vi "PicoScope6000aSettings.vi"(0 "handle in":i16, 1 "Device Info":T3, 2 "Channels":T2 {"Channel H Settings"."BandWidth" items=["Full", "100kHz", "20kHz", "1MHz", "20MHz", "25MHz", "50MHz", "200MHz", "250MHz", "500MHz"]; "Channel H Settings"."Range" items=["10mV", "20mV", "50mV", "100mV", "200mV", "500mV", "1V", "2V", "5V", "10V", "20V", "50V", "100V", "200V", "x10_Probe_100mV", "x10_Probe_200mV", "x10_Probe_500mV", "x10_Probe_1V", "x10_Probe_2V", "x10_Probe_5V", "x10_Probe_10V", "x10_Probe_20V", "x10_Probe_50V", "x10_Probe_100V", "x10_Probe_200V", "x10_Probe_500V", "CURRENT_CLAMP_60A_2A", "CURRENT_CLAMP_60A_5A", "CURRENT_CLAMP_60A_10A", "CURRENT_CLAMP_60A_20A", "CURRENT_CLAMP_60A_50A", "CURRENT_CLAMP_60A_60A", "CURRENT_CLAMP_60A_V2_0_5A", "CURRENT_CLAMP_60A_V2_1A", "CURRENT_CLAMP_60A_V2_2A", "CURRENT_CLAMP_60A_V2_5A", "CURRENT_CLAMP_60A_V2_10A", "CURRENT_CLAMP_60A_V2_20A", "CURRENT_CLAMP_60A_V2_50A", "CURRENT_CLAMP_60A_V2_60A", "RESISTANCE_LEAD_NEG5_TO_20OHM", "RESISTANCE_LEAD_NEG50_TO_200OHM", "RESISTANCE_LEAD_NEG500_TO_2KOHM", "RESISTANCE_LEAD_NEG5K_TO_20KOHM", "RESISTANCE_LEAD_NEG50K_TO_LEAD_200KOHM", "RESISTANCE_LEAD_NEG500K_TO_LEAD_2MOHM", "RESISTANCE_LEAD_DIODE_TEST", "HT_NEG3_TO_5KV", "HT_NEG3_TO_10KV", "HT_NEG5_TO_20KV", "HT_NEG5_TO_50KV", "HT_NEG5_TO_100KV", "HT_NEG3_TO_5KV_INVERTED", "HT_NEG3_TO_10KV_INVERTED", "HT_NEG5_TO_20KV_INVERTED", "HT_NEG5_TO_50KV_INVERTED", "HT_NEG5_TO_100KV_INVERTED", "TEMPERATURE_NEG50_TO_150DEGC", "PRESSURE_SENSOR_-100k-150k_PASCALS", "PRESSURE_SENSOR_-100k_TO_400k_PASCALS", "PRESSURE_SENSOR_-200k_TO_800k_PASCALS", "PRESSURE_SENSOR_-400k_TO_1600k_PASCALS", "PRESSURE_SENSOR_-400k_TO_3400k_PASCALS", "PRESSURE_SENSOR_-150k_TO_1350k_PASCALS"]; "Channel H Settings"."Coupling" items=["AC", "DC 1M Ohm", "DC 50 Ohm"]; "Channel G Settings"."BandWidth" items=["Full", "100kHz", "20kHz", "1MHz", "20MHz", "25MHz", "50MHz", "200MHz", "250MHz", "500MHz"]; "Channel G Settings"."Range" items=["10mV", "20mV", "50mV", "100mV", "200mV", "500mV", "1V", "2V", "5V", "10V", "20V", "50V", "100V", "200V", "x10_Probe_100mV", "x10_Probe_200mV", "x10_Probe_500mV", "x10_Probe_1V", "x10_Probe_2V", "x10_Probe_5V", "x10_Probe_10V", "x10_Probe_20V", "x10_Probe_50V", "x10_Probe_100V", "x10_Probe_200V", "x10_Probe_500V", "CURRENT_CLAMP_60A_2A", "CURRENT_CLAMP_60A_5A", "CURRENT_CLAMP_60A_10A", "CURRENT_CLAMP_60A_20A", "CURRENT_CLAMP_60A_50A", "CURRENT_CLAMP_60A_60A", "CURRENT_CLAMP_60A_V2_0_5A", "CURRENT_CLAMP_60A_V2_1A", "CURRENT_CLAMP_60A_V2_2A", "CURRENT_CLAMP_60A_V2_5A", "CURRENT_CLAMP_60A_V2_10A", "CURRENT_CLAMP_60A_V2_20A", "CURRENT_CLAMP_60A_V2_50A", "CURRENT_CLAMP_60A_V2_60A", "RESISTANCE_LEAD_NEG5_TO_20OHM", "RESISTANCE_LEAD_NEG50_TO_200OHM", "RESISTANCE_LEAD_NEG500_TO_2KOHM", "RESISTANCE_LEAD_NEG5K_TO_20KOHM", "RESISTANCE_LEAD_NEG50K_TO_LEAD_200KOHM", "RESISTANCE_LEAD_NEG500K_TO_LEAD_2MOHM", "RESISTANCE_LEAD_DIODE_TEST", "HT_NEG3_TO_5KV", "HT_NEG3_TO_10KV", "HT_NEG5_TO_20KV", "HT_NEG5_TO_50KV", "HT_NEG5_TO_100KV", "HT_NEG3_TO_5KV_INVERTED", "HT_NEG3_TO_10KV_INVERTED", "HT_NEG5_TO_20KV_INVERTED", "HT_NEG5_TO_50KV_INVERTED", "HT_NEG5_TO_100KV_INVERTED", "TEMPERATURE_NEG50_TO_150DEGC", "PRESSURE_SENSOR_-100k-150k_PASCALS", "PRESSURE_SENSOR_-100k_TO_400k_PASCALS", "PRESSURE_SENSOR_-200k_TO_800k_PASCALS", "PRESSURE_SENSOR_-400k_TO_1600k_PASCALS", "PRESSURE_SENSOR_-400k_TO_3400k_PASCALS", "PRESSURE_SENSOR_-150k_TO_1350k_PASCALS"]; "Channel G Settings"."Coupling" items=["AC", "DC 1M Ohm", "DC 50 Ohm"]; "Channel F Settings"."BandWidth" items=["Full", "100kHz", "20kHz", "1MHz", "20MHz", "25MHz", "50MHz", "200MHz", "250MHz", "500MHz"]; "Channel F Settings"."Range" items=["10mV", "20mV", "50mV", "100mV", "200mV", "500mV", "1V", "2V", "5V", "10V", "20V", "50V", "100V", "200V", "x10_Probe_100mV", "x10_Probe_200mV", "x10_Probe_500mV", "x10_Probe_1V", "x10_Probe_2V", "x10_Probe_5V", "x10_Probe_10V", "x10_Probe_20V", "x10_Probe_50V", "x10_Probe_100V", "x10_Probe_200V", "x10_Probe_500V", "CURRENT_CLAMP_60A_2A", "CURRENT_CLAMP_60A_5A", "CURRENT_CLAMP_60A_10A", "CURRENT_CLAMP_60A_20A", "CURRENT_CLAMP_60A_50A", "CURRENT_CLAMP_60A_60A", "CURRENT_CLAMP_60A_V2_0_5A", "CURRENT_CLAMP_60A_V2_1A", "CURRENT_CLAMP_60A_V2_2A", "CURRENT_CLAMP_60A_V2_5A", "CURRENT_CLAMP_60A_V2_10A", "CURRENT_CLAMP_60A_V2_20A", "CURRENT_CLAMP_60A_V2_50A", "CURRENT_CLAMP_60A_V2_60A", "RESISTANCE_LEAD_NEG5_TO_20OHM", "RESISTANCE_LEAD_NEG50_TO_200OHM", "RESISTANCE_LEAD_NEG500_TO_2KOHM", "RESISTANCE_LEAD_NEG5K_TO_20KOHM", "RESISTANCE_LEAD_NEG50K_TO_LEAD_200KOHM", "RESISTANCE_LEAD_NEG500K_TO_LEAD_2MOHM", "RESISTANCE_LEAD_DIODE_TEST", "HT_NEG3_TO_5KV", "HT_NEG3_TO_10KV", "HT_NEG5_TO_20KV", "HT_NEG5_TO_50KV", "HT_NEG5_TO_100KV", "HT_NEG3_TO_5KV_INVERTED", "HT_NEG3_TO_10KV_INVERTED", "HT_NEG5_TO_20KV_INVERTED", "HT_NEG5_TO_50KV_INVERTED", "HT_NEG5_TO_100KV_INVERTED", "TEMPERATURE_NEG50_TO_150DEGC", "PRESSURE_SENSOR_-100k-150k_PASCALS", "PRESSURE_SENSOR_-100k_TO_400k_PASCALS", "PRESSURE_SENSOR_-200k_TO_800k_PASCALS", "PRESSURE_SENSOR_-400k_TO_1600k_PASCALS", "PRESSURE_SENSOR_-400k_TO_3400k_PASCALS", "PRESSURE_SENSOR_-150k_TO_1350k_PASCALS"]; "Channel F Settings"."Coupling" items=["AC", "DC 1M Ohm", "DC 50 Ohm"]; "Channel E Settings"."BandWidth" items=["Full", "100kHz", "20kHz", "1MHz", "20MHz", "25MHz", "50MHz", "200MHz", "250MHz", "500MHz"]; "Channel E Settings"."Range" items=["10mV", "20mV", "50mV", "100mV", "200mV", "500mV", "1V", "2V", "5V", "10V", "20V", "50V", "100V", "200V", "x10_Probe_100mV", "x10_Probe_200mV", "x10_Probe_500mV", "x10_Probe_1V", "x10_Probe_2V", "x10_Probe_5V", "x10_Probe_10V", "x10_Probe_20V", "x10_Probe_50V", "x10_Probe_100V", "x10_Probe_200V", "x10_Probe_500V", "CURRENT_CLAMP_60A_2A", "CURRENT_CLAMP_60A_5A", "CURRENT_CLAMP_60A_10A", "CURRENT_CLAMP_60A_20A", "CURRENT_CLAMP_60A_50A", "CURRENT_CLAMP_60A_60A", "CURRENT_CLAMP_60A_V2_0_5A", "CURRENT_CLAMP_60A_V2_1A", "CURRENT_CLAMP_60A_V2_2A", "CURRENT_CLAMP_60A_V2_5A", "CURRENT_CLAMP_60A_V2_10A", "CURRENT_CLAMP_60A_V2_20A", "CURRENT_CLAMP_60A_V2_50A", "CURRENT_CLAMP_60A_V2_60A", "RESISTANCE_LEAD_NEG5_TO_20OHM", "RESISTANCE_LEAD_NEG50_TO_200OHM", "RESISTANCE_LEAD_NEG500_TO_2KOHM", "RESISTANCE_LEAD_NEG5K_TO_20KOHM", "RESISTANCE_LEAD_NEG50K_TO_LEAD_200KOHM", "RESISTANCE_LEAD_NEG500K_TO_LEAD_2MOHM", "RESISTANCE_LEAD_DIODE_TEST", "HT_NEG3_TO_5KV", "HT_NEG3_TO_10KV", "HT_NEG5_TO_20KV", "HT_NEG5_TO_50KV", "HT_NEG5_TO_100KV", "HT_NEG3_TO_5KV_INVERTED", "HT_NEG3_TO_10KV_INVERTED", "HT_NEG5_TO_20KV_INVERTED", "HT_NEG5_TO_50KV_INVERTED", "HT_NEG5_TO_100KV_INVERTED", "TEMPERATURE_NEG50_TO_150DEGC", "PRESSURE_SENSOR_-100k-150k_PASCALS", "PRESSURE_SENSOR_-100k_TO_400k_PASCALS", "PRESSURE_SENSOR_-200k_TO_800k_PASCALS", "PRESSURE_SENSOR_-400k_TO_1600k_PASCALS", "PRESSURE_SENSOR_-400k_TO_3400k_PASCALS", "PRESSURE_SENSOR_-150k_TO_1350k_PASCALS"]; "Channel E Settings"."Coupling" items=["AC", "DC 1M Ohm", "DC 50 Ohm"]; "Channel D Settings"."BandWidth" items=["Full", "100kHz", "20kHz", "1MHz", "20MHz", "25MHz", "50MHz", "200MHz", "250MHz", "500MHz"]; "Channel D Settings"."Range" items=["10mV", "20mV", "50mV", "100mV", "200mV", "500mV", "1V", "2V", "5V", "10V", "20V", "50V", "100V", "200V", "x10_Probe_100mV", "x10_Probe_200mV", "x10_Probe_500mV", "x10_Probe_1V", "x10_Probe_2V", "x10_Probe_5V", "x10_Probe_10V", "x10_Probe_20V", "x10_Probe_50V", "x10_Probe_100V", "x10_Probe_200V", "x10_Probe_500V", "CURRENT_CLAMP_60A_2A", "CURRENT_CLAMP_60A_5A", "CURRENT_CLAMP_60A_10A", "CURRENT_CLAMP_60A_20A", "CURRENT_CLAMP_60A_50A", "CURRENT_CLAMP_60A_60A", "CURRENT_CLAMP_60A_V2_0_5A", "CURRENT_CLAMP_60A_V2_1A", "CURRENT_CLAMP_60A_V2_2A", "CURRENT_CLAMP_60A_V2_5A", "CURRENT_CLAMP_60A_V2_10A", "CURRENT_CLAMP_60A_V2_20A", "CURRENT_CLAMP_60A_V2_50A", "CURRENT_CLAMP_60A_V2_60A", "RESISTANCE_LEAD_NEG5_TO_20OHM", "RESISTANCE_LEAD_NEG50_TO_200OHM", "RESISTANCE_LEAD_NEG500_TO_2KOHM", "RESISTANCE_LEAD_NEG5K_TO_20KOHM", "RESISTANCE_LEAD_NEG50K_TO_LEAD_200KOHM", "RESISTANCE_LEAD_NEG500K_TO_LEAD_2MOHM", "RESISTANCE_LEAD_DIODE_TEST", "HT_NEG3_TO_5KV", "HT_NEG3_TO_10KV", "HT_NEG5_TO_20KV", "HT_NEG5_TO_50KV", "HT_NEG5_TO_100KV", "HT_NEG3_TO_5KV_INVERTED", "HT_NEG3_TO_10KV_INVERTED", "HT_NEG5_TO_20KV_INVERTED", "HT_NEG5_TO_50KV_INVERTED", "HT_NEG5_TO_100KV_INVERTED", "TEMPERATURE_NEG50_TO_150DEGC", "PRESSURE_SENSOR_-100k-150k_PASCALS", "PRESSURE_SENSOR_-100k_TO_400k_PASCALS", "PRESSURE_SENSOR_-200k_TO_800k_PASCALS", "PRESSURE_SENSOR_-400k_TO_1600k_PASCALS", "PRESSURE_SENSOR_-400k_TO_3400k_PASCALS", "PRESSURE_SENSOR_-150k_TO_1350k_PASCALS"]; "Channel D Settings"."Coupling" items=["AC", "DC 1M Ohm", "DC 50 Ohm"]; "Channel C Settings"."BandWidth" items=["Full", "100kHz", "20kHz", "1MHz", "20MHz", "25MHz", "50MHz", "200MHz", "250MHz", "500MHz"]; "Channel C Settings"."Range" items=["10mV", "20mV", "50mV", "100mV", "200mV", "500mV", "1V", "2V", "5V", "10V", "20V", "50V", "100V", "200V", "x10_Probe_100mV", "x10_Probe_200mV", "x10_Probe_500mV", "x10_Probe_1V", "x10_Probe_2V", "x10_Probe_5V", "x10_Probe_10V", "x10_Probe_20V", "x10_Probe_50V", "x10_Probe_100V", "x10_Probe_200V", "x10_Probe_500V", "CURRENT_CLAMP_60A_2A", "CURRENT_CLAMP_60A_5A", "CURRENT_CLAMP_60A_10A", "CURRENT_CLAMP_60A_20A", "CURRENT_CLAMP_60A_50A", "CURRENT_CLAMP_60A_60A", "CURRENT_CLAMP_60A_V2_0_5A", "CURRENT_CLAMP_60A_V2_1A", "CURRENT_CLAMP_60A_V2_2A", "CURRENT_CLAMP_60A_V2_5A", "CURRENT_CLAMP_60A_V2_10A", "CURRENT_CLAMP_60A_V2_20A", "CURRENT_CLAMP_60A_V2_50A", "CURRENT_CLAMP_60A_V2_60A", "RESISTANCE_LEAD_NEG5_TO_20OHM", "RESISTANCE_LEAD_NEG50_TO_200OHM", "RESISTANCE_LEAD_NEG500_TO_2KOHM", "RESISTANCE_LEAD_NEG5K_TO_20KOHM", "RESISTANCE_LEAD_NEG50K_TO_LEAD_200KOHM", "RESISTANCE_LEAD_NEG500K_TO_LEAD_2MOHM", "RESISTANCE_LEAD_DIODE_TEST", "HT_NEG3_TO_5KV", "HT_NEG3_TO_10KV", "HT_NEG5_TO_20KV", "HT_NEG5_TO_50KV", "HT_NEG5_TO_100KV", "HT_NEG3_TO_5KV_INVERTED", "HT_NEG3_TO_10KV_INVERTED", "HT_NEG5_TO_20KV_INVERTED", "HT_NEG5_TO_50KV_INVERTED", "HT_NEG5_TO_100KV_INVERTED", "TEMPERATURE_NEG50_TO_150DEGC", "PRESSURE_SENSOR_-100k-150k_PASCALS", "PRESSURE_SENSOR_-100k_TO_400k_PASCALS", "PRESSURE_SENSOR_-200k_TO_800k_PASCALS", "PRESSURE_SENSOR_-400k_TO_1600k_PASCALS", "PRESSURE_SENSOR_-400k_TO_3400k_PASCALS", "PRESSURE_SENSOR_-150k_TO_1350k_PASCALS"]; "Channel C Settings"."Coupling" items=["AC", "DC 1M Ohm", "DC 50 Ohm"]; "Channel B Settings"."BandWidth" items=["Full", "100kHz", "20kHz", "1MHz", "20MHz", "25MHz", "50MHz", "200MHz", "250MHz", "500MHz"]; "Channel B Settings"."Range" items=["10mV", "20mV", "50mV", "100mV", "200mV", "500mV", "1V", "2V", "5V", "10V", "20V", "50V", "100V", "200V", "x10_Probe_100mV", "x10_Probe_200mV", "x10_Probe_500mV", "x10_Probe_1V", "x10_Probe_2V", "x10_Probe_5V", "x10_Probe_10V", "x10_Probe_20V", "x10_Probe_50V", "x10_Probe_100V", "x10_Probe_200V", "x10_Probe_500V", "CURRENT_CLAMP_60A_2A", "CURRENT_CLAMP_60A_5A", "CURRENT_CLAMP_60A_10A", "CURRENT_CLAMP_60A_20A", "CURRENT_CLAMP_60A_50A", "CURRENT_CLAMP_60A_60A", "CURRENT_CLAMP_60A_V2_0_5A", "CURRENT_CLAMP_60A_V2_1A", "CURRENT_CLAMP_60A_V2_2A", "CURRENT_CLAMP_60A_V2_5A", "CURRENT_CLAMP_60A_V2_10A", "CURRENT_CLAMP_60A_V2_20A", "CURRENT_CLAMP_60A_V2_50A", "CURRENT_CLAMP_60A_V2_60A", "RESISTANCE_LEAD_NEG5_TO_20OHM", "RESISTANCE_LEAD_NEG50_TO_200OHM", "RESISTANCE_LEAD_NEG500_TO_2KOHM", "RESISTANCE_LEAD_NEG5K_TO_20KOHM", "RESISTANCE_LEAD_NEG50K_TO_LEAD_200KOHM", "RESISTANCE_LEAD_NEG500K_TO_LEAD_2MOHM", "RESISTANCE_LEAD_DIODE_TEST", "HT_NEG3_TO_5KV", "HT_NEG3_TO_10KV", "HT_NEG5_TO_20KV", "HT_NEG5_TO_50KV", "HT_NEG5_TO_100KV", "HT_NEG3_TO_5KV_INVERTED", "HT_NEG3_TO_10KV_INVERTED", "HT_NEG5_TO_20KV_INVERTED", "HT_NEG5_TO_50KV_INVERTED", "HT_NEG5_TO_100KV_INVERTED", "TEMPERATURE_NEG50_TO_150DEGC", "PRESSURE_SENSOR_-100k-150k_PASCALS", "PRESSURE_SENSOR_-100k_TO_400k_PASCALS", "PRESSURE_SENSOR_-200k_TO_800k_PASCALS", "PRESSURE_SENSOR_-400k_TO_1600k_PASCALS", "PRESSURE_SENSOR_-400k_TO_3400k_PASCALS", "PRESSURE_SENSOR_-150k_TO_1350k_PASCALS"]; "Channel B Settings"."Coupling" items=["AC", "DC 1M Ohm", "DC 50 Ohm"]; "Channel A Settings"."Range" items=["10mV", "20mV", "50mV", "100mV", "200mV", "500mV", "1V", "2V", "5V", "10V", "20V", "50V", "100V", "200V", "x10_Probe_100mV", "x10_Probe_200mV", "x10_Probe_500mV", "x10_Probe_1V", "x10_Probe_2V", "x10_Probe_5V", "x10_Probe_10V", "x10_Probe_20V", "x10_Probe_50V", "x10_Probe_100V", "x10_Probe_200V", "x10_Probe_500V", "CURRENT_CLAMP_60A_2A", "CURRENT_CLAMP_60A_5A", "CURRENT_CLAMP_60A_10A", "CURRENT_CLAMP_60A_20A", "CURRENT_CLAMP_60A_50A", "CURRENT_CLAMP_60A_60A", "CURRENT_CLAMP_60A_V2_0_5A", "CURRENT_CLAMP_60A_V2_1A", "CURRENT_CLAMP_60A_V2_2A", "CURRENT_CLAMP_60A_V2_5A", "CURRENT_CLAMP_60A_V2_10A", "CURRENT_CLAMP_60A_V2_20A", "CURRENT_CLAMP_60A_V2_50A", "CURRENT_CLAMP_60A_V2_60A", "RESISTANCE_LEAD_NEG5_TO_20OHM", "RESISTANCE_LEAD_NEG50_TO_200OHM", "RESISTANCE_LEAD_NEG500_TO_2KOHM", "RESISTANCE_LEAD_NEG5K_TO_20KOHM", "RESISTANCE_LEAD_NEG50K_TO_LEAD_200KOHM", "RESISTANCE_LEAD_NEG500K_TO_LEAD_2MOHM", "RESISTANCE_LEAD_DIODE_TEST", "HT_NEG3_TO_5KV", "HT_NEG3_TO_10KV", "HT_NEG5_TO_20KV", "HT_NEG5_TO_50KV", "HT_NEG5_TO_100KV", "HT_NEG3_TO_5KV_INVERTED", "HT_NEG3_TO_10KV_INVERTED", "HT_NEG5_TO_20KV_INVERTED", "HT_NEG5_TO_50KV_INVERTED", "HT_NEG5_TO_100KV_INVERTED", "TEMPERATURE_NEG50_TO_150DEGC", "PRESSURE_SENSOR_-100k-150k_PASCALS", "PRESSURE_SENSOR_-100k_TO_400k_PASCALS", "PRESSURE_SENSOR_-200k_TO_800k_PASCALS", "PRESSURE_SENSOR_-400k_TO_1600k_PASCALS", "PRESSURE_SENSOR_-400k_TO_3400k_PASCALS", "PRESSURE_SENSOR_-150k_TO_1350k_PASCALS"]; "Channel A Settings"."BandWidth" items=["Full", "100kHz", "20kHz", "1MHz", "20MHz", "25MHz", "50MHz", "200MHz", "250MHz", "500MHz"]; "Channel A Settings"."Coupling" items=["AC", "DC 1M Ohm", "DC 50 Ohm"]}, 7 "Max ADC value":i16, 11 "error in (no error)":errorcluster, 12 "Trigger Settings":T4 {"Trigger Source" items=["Channel A", "Channel B", "Channel C", "Channel D", "Channel E", "Channel F", "Channel G", "Channel H", "Port 0", "Port 1", "Trigger AUX"]; "Trigger Direction" items=["Above", "Below", "Rising", "Falling", "Rising or Falling"]; "Trigger Threshold (Volts/Probe Units)" format="%#_6p"}, 14 "Digital Channels":T1 {"Port 1 Settings"."Threshold Level (Volts)" format="%#_4p"; "Port 1 Settings"."Hysteresis" items=["PICO_VERY_HIGH_400MV", "PICO_HIGH_200MV", "PICO_NORMAL_100MV", "PICO_LOW_50MV"]; "Port 0 Settings"."Threshold Level (Volts)" format="%#_4p"; "Port 0 Settings"."Hysteresis" items=["PICO_VERY_HIGH_400MV", "PICO_HIGH_200MV", "PICO_NORMAL_100MV", "PICO_LOW_50MV"]}) -> (3 "Enabled array":i16[](array[numeric]), 4 "handle out":i16, 15 "error out":errorcluster)   [LabVIEW 2009]
doc: "Sets up channels and calls setSimpleTrigger"
uses:
  ps6000a.dll
  PicoScope6000aAnalogChannelSettings.ctl
  PicoScope6000aDigitalChannelSettings.ctl
panel:
  # "D8-D15"
  # "DO-D7"
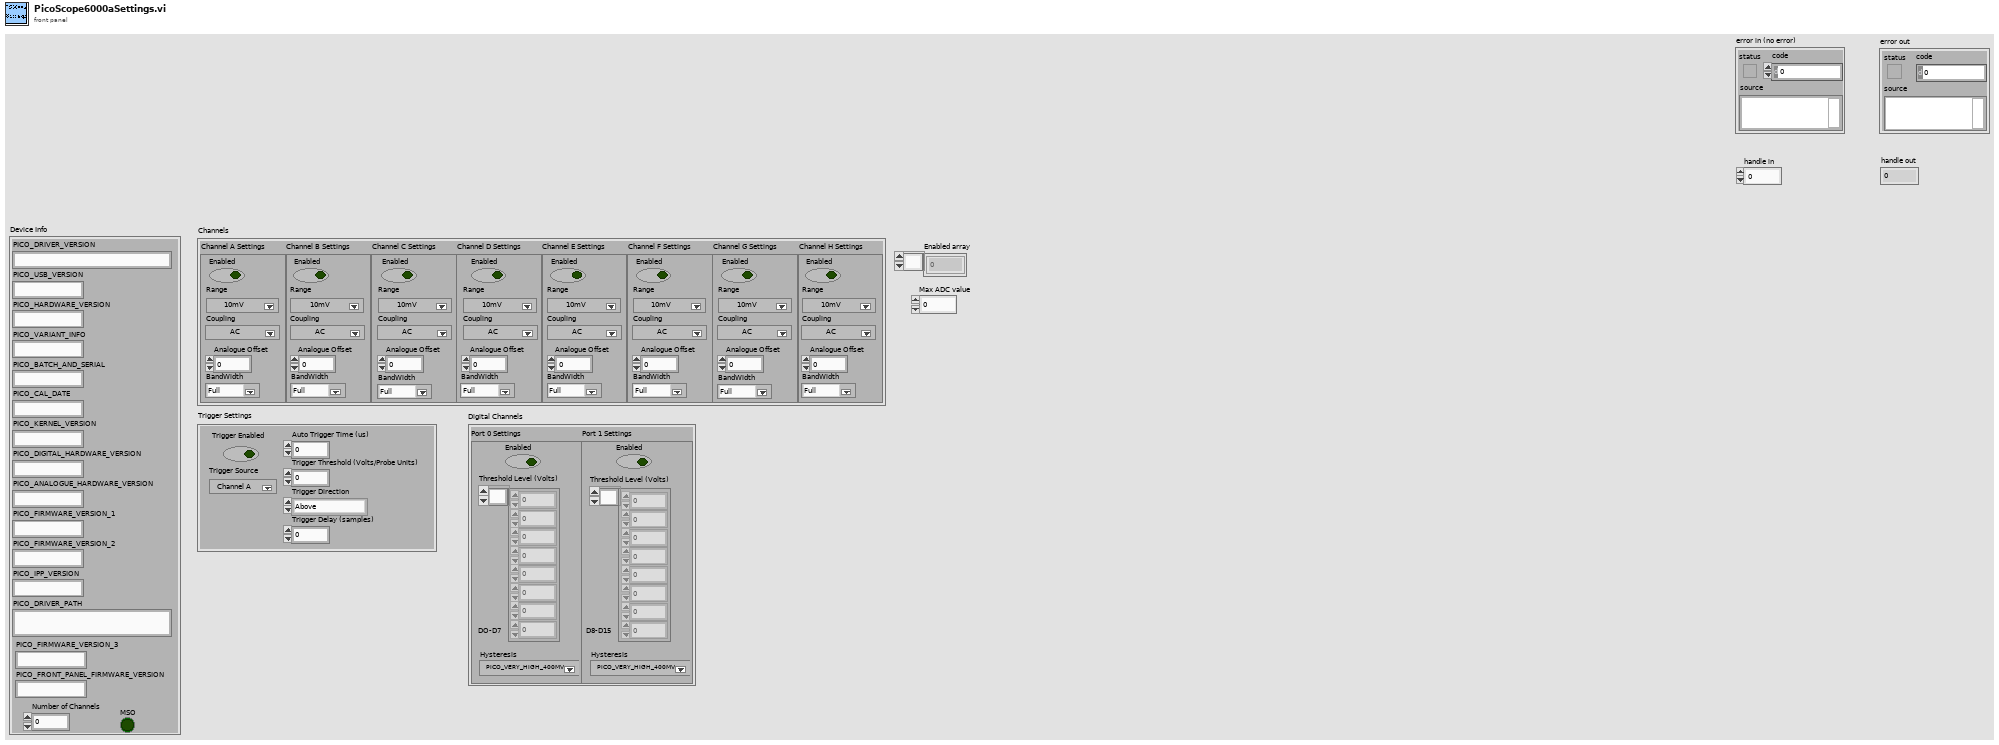
[diagram p1: front panel]
types:
  T1 = typedef "PicoScope6000aDigitalChannelSettings.ctl" = cluster{"Port 0 Settings ":cluster{"Enabled":bool, "Hysteresis":u32, "Threshold Level (Volts)":dbl[]}, "Port 1 Settings":cluster{"Enabled":bool, "Hysteresis":u32, "Threshold Level (Volts)":dbl[]}}
  T2 = typedef "PicoScope6000aAnalogChannelSettings.ctl" = cluster{"Channel A Settings ":cluster{"Enabled":bool, "Coupling":i16, "Range":u16, "Analogue Offset":dbl, "BandWidth":u32}, "Channel B Settings ":cluster{"Enabled":bool, "Coupling":i16, "Range":u16, "Analogue Offset":dbl, "BandWidth":u32}, "Channel C Settings ":cluster{"Enabled":bool, "Coupling":i16, "Range":u16, "Analogue Offset":dbl, "BandWidth":u32}, "Channel D Settings ":cluster{"Enabled":bool, "Coupling":i16, "Range":u16, "Analogue Offset":dbl, "BandWidth":u32}, "Channel E Settings ":cluster{"Enabled":bool, "Coupling":i16, "Range":u16, "Analogue Offset":dbl, "BandWidth":u32}, "Channel F Settings ":cluster{"Enabled":bool, "Coupling":i16, "Range":u16, "Analogue Offset":dbl, "BandWidth":u32}, "Channel G Settings ":cluster{"Enabled":bool, "Coupling":i16, "Range":u16, "Analogue Offset":dbl, "BandWidth":u32}, "Channel H Settings ":cluster{"Enabled":bool, "Coupling":i16, "Range":u16, "Analogue Offset":dbl, "BandWidth":u32}}
  T3 = cluster{"PICO_DRIVER_VERSION":string, "PICO_USB_VERSION":string, "PICO_HARDWARE_VERSION":string, "PICO_VARIANT_INFO":string, "PICO_BATCH_AND_SERIAL":string, "PICO_CAL_DATE":string, "PICO_KERNEL_VERSION":string, "PICO_DIGITAL_HARDWARE_VERSION":string, "PICO_ANALOGUE_HARDWARE_VERSION":string, "PICO_FIRMWARE_VERSION_1":string, "PICO_FIRMWARE_VERSION_2":string, "PICO_IPP_VERSION":string, "PICO_DRIVER_PATH":string, "PICO_FIRMWARE_VERSION_3":string, "PICO_FRONT_PANEL_FIRMWARE_VERSION":string, "Number of Channels":i16, "MSO":bool}
  T4 = cluster{"Trigger Enabled":bool, "Trigger Threshold (Volts/Probe Units)":dbl, "Trigger Direction":u16, "Trigger Delay (samples)":u64, "Auto Trigger Time (us)":u32, "Trigger Source":u32}
  T5 = cluster{"Enabled":bool, "Coupling":i16, "Range":u16, "Analogue Offset":dbl, "BandWidth":u32}
  T6 = cluster{"Enabled":bool, "Hysteresis":u32, "Threshold Level (Volts)":dbl[]}
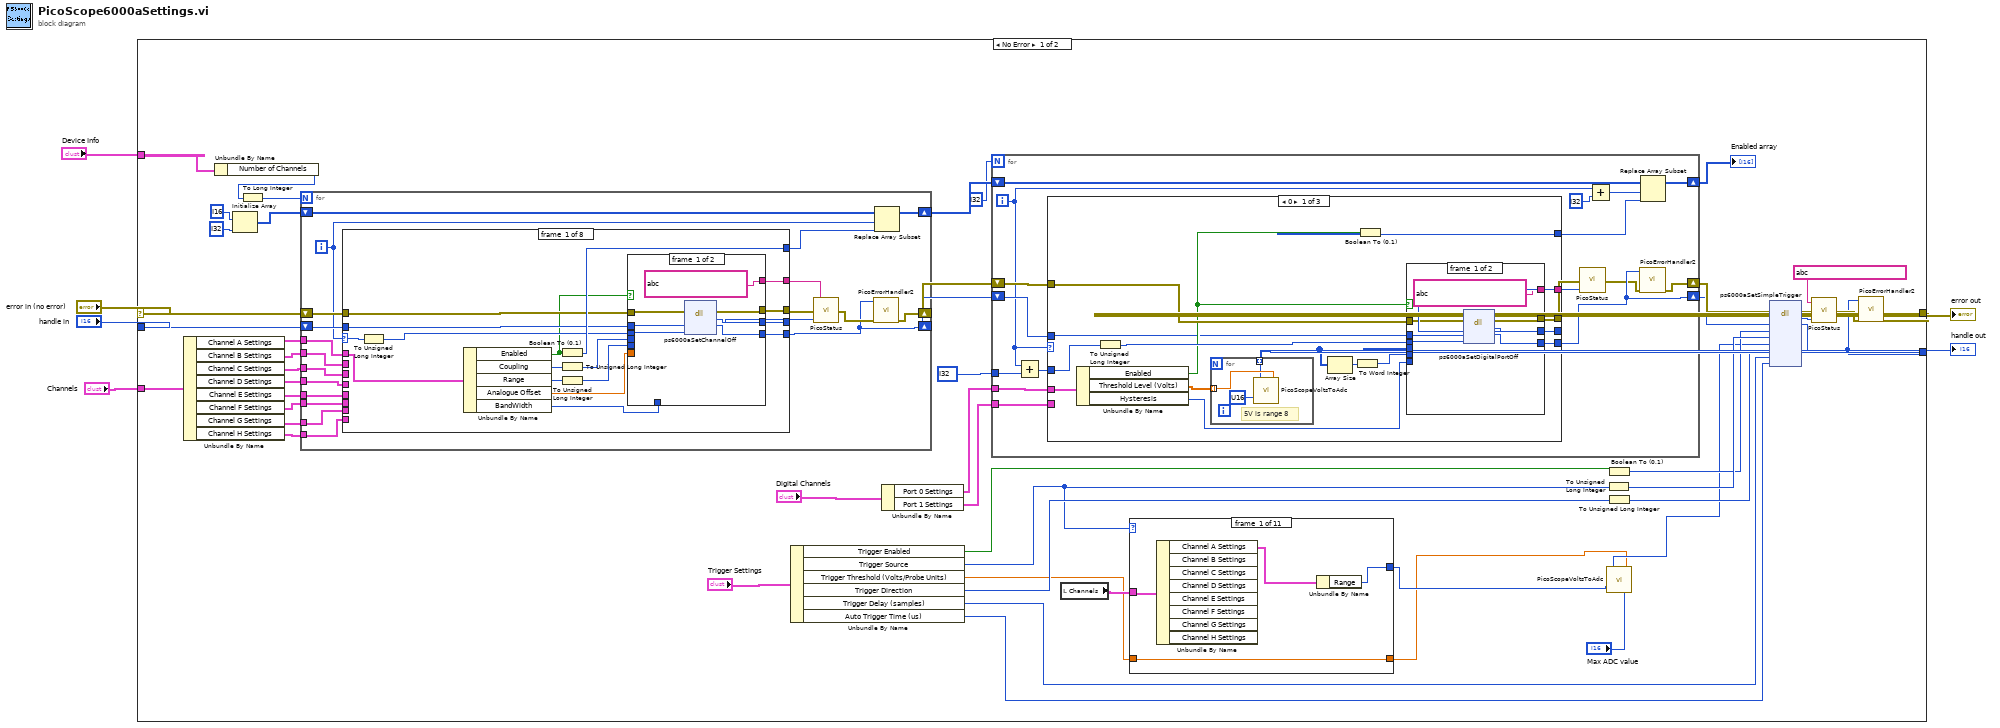
[diagram p0: block diagram]
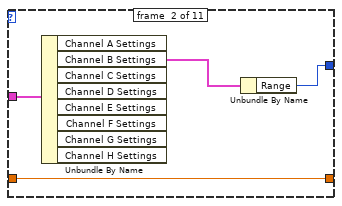
[diagram p2: hidden frame]
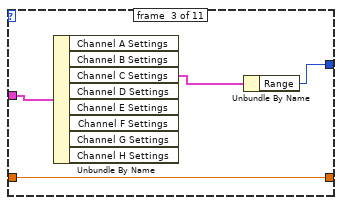
[diagram p3: hidden frame]
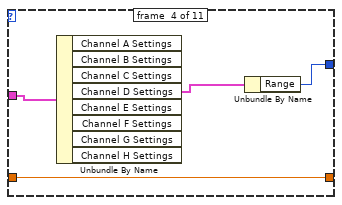
[diagram p4: hidden frame]
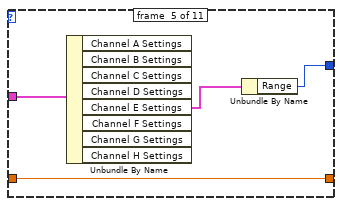
[diagram p5: hidden frame]
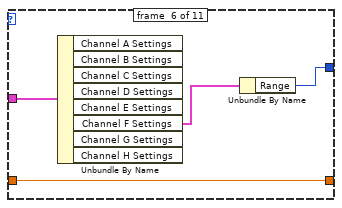
[diagram p6: hidden frame]
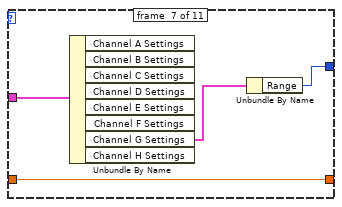
[diagram p7: hidden frame]
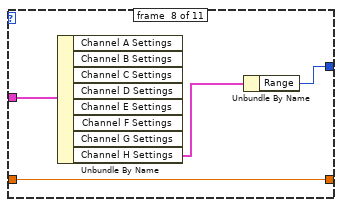
[diagram p8: hidden frame]
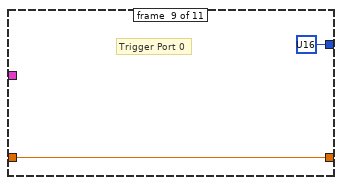
[diagram p9: hidden frame]
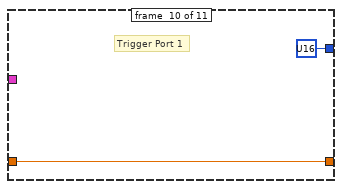
[diagram p10: hidden frame]
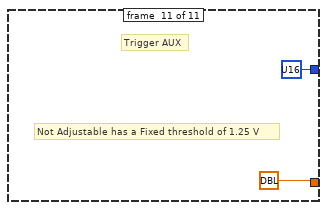
[diagram p11: hidden frame]
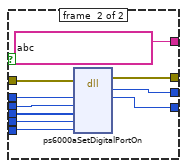
[diagram p12: hidden frame]
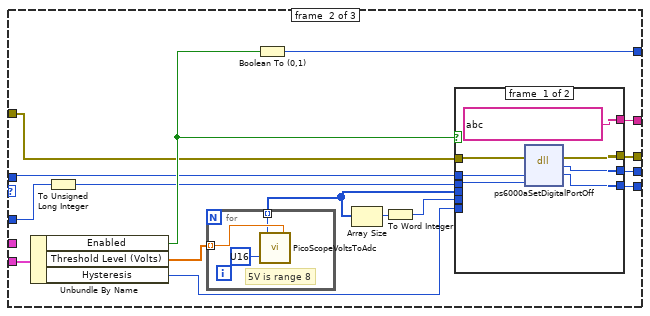
[diagram p13: hidden frame]
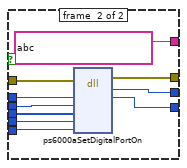
[diagram p14: hidden frame]
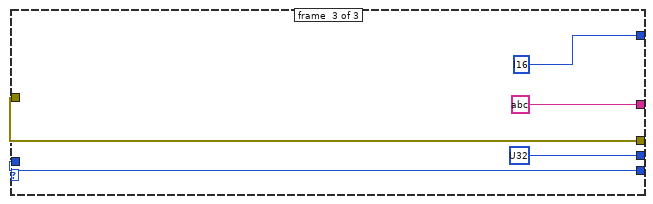
[diagram p15: hidden frame]
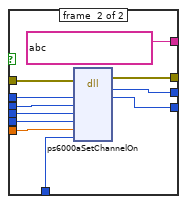
[diagram p16: hidden frame]
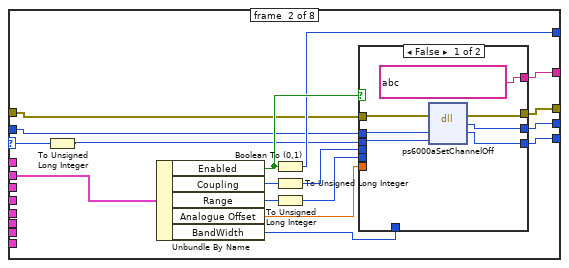
[diagram p17: hidden frame]
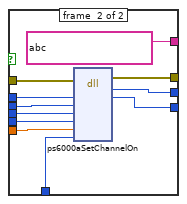
[diagram p18: hidden frame]
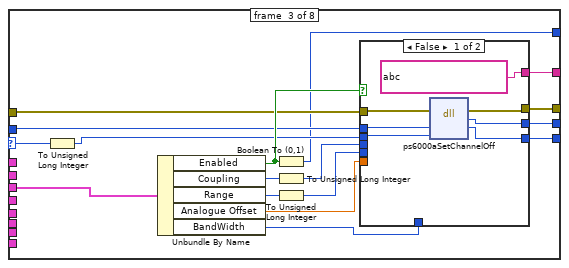
[diagram p19: hidden frame]
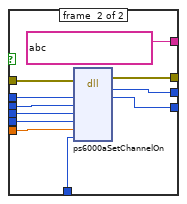
[diagram p20: hidden frame]
diagram:
  n1 = case shown="No Error" "error in (no error)" {
    selector: "error in (no error)" -> [w43 w490]
    tunnel: "handle in" -> [w44 w489]
    tunnel: [w34 w489] -> w6
    tunnel: [w36 w490] -> w5
    tunnel: "Device Info" -> [w39 _]
    tunnel: "Channels" -> [w25 _]
    frame #0 {
      n2 = Unbundle By Name(w25) -> ("Channel A Settings"=w32:T5, "Channel B Settings"=w33:T5, "Channel C Settings"=w31:T5, "Channel D Settings"=w30:T5, "Channel E Settings"=w29:T5, "Channel F Settings"=w26:T5, "Channel G Settings"=w27:T5, "Channel H Settings"=w28:T5)
      n3 = Unbundle By Name(w39) -> ("Number of Channels"=w38:i16)
      n4 = Initialize Array(i16 ? ("element"), i32 ? ("dimension size")) -> (w40:i16[])
      n5 = To Long Integer(number=w38) -> (32bit integer=w37:i32)
      n6 = for {
        N: w37 -> [_]
        shift-right: [w202] -> w20
        shift-left: w43 -> [w207]
        shift-right: [w197] -> w19
        shift-left: w44 -> [w208]
        shift-right: [w203] -> w23
        shift-left: w40 -> [w204]
        tunnel: w33 -> [w196]
        tunnel: w32 -> [w195]
        tunnel: w31 -> [w194]
        tunnel: w30 -> [w193]
        tunnel: w29 -> [w192]
        tunnel: w28 -> [w191]
        tunnel: w27 -> [w190]
        tunnel: w26 -> [w189]
        i -> [w206]
        n7 = case shown="3" w206 {
          selector: w206 -> [w225 w260 w295 w330 w365 w400 w435 w470]
          tunnel: w208 -> [w218 w251 w286 w318 w356 w392 w427 w457]
          tunnel: w207 -> [w220 w252 w287 w323 w357 w391 w426 w458]
          tunnel: [w222 w253 w285 w316 w358 w390 w425 w463] -> w205
          tunnel: [w212 w248 w282 w321 w352 w387 w422 w460] -> w201
          tunnel: [w219 w247 w283 w322 w353 w388 w423 w461] -> w200
          tunnel: [w221 w246 w284 w319 w354 w389 w424 w462] -> w199
          tunnel: [w211 w249 w281 w320 w351 w386 w421 w459] -> w197
          tunnel: w196 -> [_ w245 _ _ _ _ _ _]
          tunnel: w195 -> [w210 _ _ _ _ _ _ _]
          tunnel: w194 -> [_ _ w280 _ _ _ _ _]
          tunnel: w193 -> [_ _ _ w315 _ _ _ _]
          tunnel: w192 -> [_ _ _ _ w350 _ _ _]
          tunnel: w191 -> [_ _ _ _ _ _ _ w455]
          tunnel: w190 -> [_ _ _ _ _ _ w420 _]
          tunnel: w189 -> [_ _ _ _ _ w385 _ _]
          frame #0 {
            n8 = To Unsigned Long Integer(number=w225) -> (unsigned 32bit integer=w217:u32)
            n9 = Unbundle By Name(w210) -> ("Enabled"=w213:bool, "Coupling"=w224:i16, "Range"=w223:u16, "Analogue Offset"=w214:dbl, "BandWidth"=w209:u32)
            n10 = Boolean To (0,1)(Boolean=w213) -> (0, 1=w222:i16)
            n11 = To Unsigned Long Integer(number=w224) -> (unsigned 32bit integer=w216:u32)
            n12 = To Unsigned Long Integer(number=w223) -> (unsigned 32bit integer=w215:u32)
            n13 = case shown="True" w213 {
              tunnel: [string ? ("source") string ? ("source")] -> w221
              tunnel: w220 -> [w231 w242]
              tunnel: [w230 w241] -> w219
              tunnel: w218 -> [w229 w240]
              tunnel: w217 -> [w228 w239]
              tunnel: w216 -> [_ w238]
              tunnel: w215 -> [_ w237]
              tunnel: w214 -> [_ w236]
              tunnel: [w227 w235] -> w212
              tunnel: [w226 w234] -> w211
              tunnel: w209 -> [_ w233]
              frame #0 {
                n14 = dll-call lib="ps6000a.dll" fn="ps6000aSetChannelOff" ("ps3000.dll:_ps3000_open_unit@0")(error in=w231, "handle"=w229, "channel"=w228) -> (error out=w230:errorcluster, "PICO_STATUS"=w227:u32, "handle"=w226:i16)  [unwired: 3 in, 1 out]
              }
              frame #1 {
                n15 = dll-call lib="ps6000a.dll" fn="ps6000aSetChannelOn" ("ps3000.dll:_ps3000_open_unit@0")(error in=w242, "handle"=w240, "channel"=w239, "coupling"=w238, "range"=w237, "analogueOffset"=w236, "bandwidth"=w233) -> (error out=w241:errorcluster, "PICO_STATUS"=w235:u32, "handle"=w234:i16)  [unwired: 7 in, 1 out]
              }
            }
          }
          frame #1 {
            n16 = To Unsigned Long Integer(number=w260) -> (unsigned 32bit integer=w250:u32)
            n17 = Unbundle By Name(w245) -> ("Enabled"=w254:bool, "Coupling"=w259:i16, "Range"=w258:u16, "Analogue Offset"=w255:dbl, "BandWidth"=w244:u32)
            n18 = Boolean To (0,1)(Boolean=w254) -> (0, 1=w253:i16)
            n19 = To Unsigned Long Integer(number=w259) -> (unsigned 32bit integer=w257:u32)
            n20 = To Unsigned Long Integer(number=w258) -> (unsigned 32bit integer=w256:u32)
            n21 = case shown="False" w254 {
              tunnel: [string ? ("source") string ? ("source")] -> w246
              tunnel: w252 -> [w266 w277]
              tunnel: [w265 w276] -> w247
              tunnel: w251 -> [w264 w275]
              tunnel: w250 -> [w263 w274]
              tunnel: w257 -> [_ w273]
              tunnel: w256 -> [_ w272]
              tunnel: w255 -> [_ w271]
              tunnel: [w262 w270] -> w248
              tunnel: [w261 w269] -> w249
              tunnel: w244 -> [_ w268]
              frame #0 {
                n22 = dll-call lib="ps6000a.dll" fn="ps6000aSetChannelOff" ("ps3000.dll:_ps3000_open_unit@0")(error in=w266, "handle"=w264, "channel"=w263) -> (error out=w265:errorcluster, "PICO_STATUS"=w262:u32, "handle"=w261:i16)  [unwired: 3 in, 1 out]
              }
              frame #1 {
                n23 = dll-call lib="ps6000a.dll" fn="ps6000aSetChannelOn" ("ps3000.dll:_ps3000_open_unit@0")(error in=w277, "handle"=w275, "channel"=w274, "coupling"=w273, "range"=w272, "analogueOffset"=w271, "bandwidth"=w268) -> (error out=w276:errorcluster, "PICO_STATUS"=w270:u32, "handle"=w269:i16)  [unwired: 7 in, 1 out]
              }
            }
          }
          frame #2 {
            n24 = To Unsigned Long Integer(number=w295) -> (unsigned 32bit integer=w288:u32)
            n25 = Unbundle By Name(w280) -> ("Enabled"=w294:bool, "Coupling"=w289:i16, "Range"=w290:u16, "Analogue Offset"=w293:dbl, "BandWidth"=w279:u32)
            n26 = Boolean To (0,1)(Boolean=w294) -> (0, 1=w285:i16)
            n27 = To Unsigned Long Integer(number=w289) -> (unsigned 32bit integer=w291:u32)
            n28 = To Unsigned Long Integer(number=w290) -> (unsigned 32bit integer=w292:u32)
            n29 = case shown="False" w294 {
              tunnel: [string ? ("source") string ? ("source")] -> w284
              tunnel: w287 -> [w301 w312]
              tunnel: [w300 w311] -> w283
              tunnel: w286 -> [w299 w310]
              tunnel: w288 -> [w298 w309]
              tunnel: w291 -> [_ w308]
              tunnel: w292 -> [_ w307]
              tunnel: w293 -> [_ w306]
              tunnel: [w297 w305] -> w282
              tunnel: [w296 w304] -> w281
              tunnel: w279 -> [_ w303]
              frame #0 {
                n30 = dll-call lib="ps6000a.dll" fn="ps6000aSetChannelOff" ("ps3000.dll:_ps3000_open_unit@0")(error in=w301, "handle"=w299, "channel"=w298) -> (error out=w300:errorcluster, "PICO_STATUS"=w297:u32, "handle"=w296:i16)  [unwired: 3 in, 1 out]
              }
              frame #1 {
                n31 = dll-call lib="ps6000a.dll" fn="ps6000aSetChannelOn" ("ps3000.dll:_ps3000_open_unit@0")(error in=w312, "handle"=w310, "channel"=w309, "coupling"=w308, "range"=w307, "analogueOffset"=w306, "bandwidth"=w303) -> (error out=w311:errorcluster, "PICO_STATUS"=w305:u32, "handle"=w304:i16)  [unwired: 7 in, 1 out]
              }
            }
          }
          frame #3 {
            n32 = To Unsigned Long Integer(number=w330) -> (unsigned 32bit integer=w317:u32)
            n33 = Unbundle By Name(w315) -> ("Enabled"=w324:bool, "Coupling"=w329:i16, "Range"=w328:u16, "Analogue Offset"=w325:dbl, "BandWidth"=w314:u32)
            n34 = Boolean To (0,1)(Boolean=w324) -> (0, 1=w316:i16)
            n35 = To Unsigned Long Integer(number=w329) -> (unsigned 32bit integer=w327:u32)
            n36 = To Unsigned Long Integer(number=w328) -> (unsigned 32bit integer=w326:u32)
            n37 = case shown="True" w324 {
              tunnel: [string ? ("source") string ? ("source")] -> w319
              tunnel: w323 -> [w336 w347]
              tunnel: [w335 w346] -> w322
              tunnel: w318 -> [w334 w345]
              tunnel: w317 -> [w333 w344]
              tunnel: w327 -> [_ w343]
              tunnel: w326 -> [_ w342]
              tunnel: w325 -> [_ w341]
              tunnel: [w332 w340] -> w321
              tunnel: [w331 w339] -> w320
              tunnel: w314 -> [_ w338]
              frame #0 {
                n38 = dll-call lib="ps6000a.dll" fn="ps6000aSetChannelOff" ("ps3000.dll:_ps3000_open_unit@0")(error in=w336, "handle"=w334, "channel"=w333) -> (error out=w335:errorcluster, "PICO_STATUS"=w332:u32, "handle"=w331:i16)  [unwired: 3 in, 1 out]
              }
              frame #1 {
                n39 = dll-call lib="ps6000a.dll" fn="ps6000aSetChannelOn" ("ps3000.dll:_ps3000_open_unit@0")(error in=w347, "handle"=w345, "channel"=w344, "coupling"=w343, "range"=w342, "analogueOffset"=w341, "bandwidth"=w338) -> (error out=w346:errorcluster, "PICO_STATUS"=w340:u32, "handle"=w339:i16)  [unwired: 7 in, 1 out]
              }
            }
          }
          frame #4 {
            n40 = To Unsigned Long Integer(number=w365) -> (unsigned 32bit integer=w355:u32)
            n41 = Unbundle By Name(w350) -> ("Enabled"=w359:bool, "Coupling"=w364:i16, "Range"=w363:u16, "Analogue Offset"=w360:dbl, "BandWidth"=w349:u32)
            n42 = Boolean To (0,1)(Boolean=w359) -> (0, 1=w358:i16)
            n43 = To Unsigned Long Integer(number=w364) -> (unsigned 32bit integer=w362:u32)
            n44 = To Unsigned Long Integer(number=w363) -> (unsigned 32bit integer=w361:u32)
            n45 = case shown="False" w359 {
              tunnel: [string ? ("source") string ? ("source")] -> w354
              tunnel: w357 -> [w371 w382]
              tunnel: [w370 w381] -> w353
              tunnel: w356 -> [w369 w380]
              tunnel: w355 -> [w368 w379]
              tunnel: w362 -> [_ w378]
              tunnel: w361 -> [_ w377]
              tunnel: w360 -> [_ w376]
              tunnel: [w367 w375] -> w352
              tunnel: [w366 w374] -> w351
              tunnel: w349 -> [_ w373]
              frame #0 {
                n46 = dll-call lib="ps6000a.dll" fn="ps6000aSetChannelOff" ("ps3000.dll:_ps3000_open_unit@0")(error in=w371, "handle"=w369, "channel"=w368) -> (error out=w370:errorcluster, "PICO_STATUS"=w367:u32, "handle"=w366:i16)  [unwired: 3 in, 1 out]
              }
              frame #1 {
                n47 = dll-call lib="ps6000a.dll" fn="ps6000aSetChannelOn" ("ps3000.dll:_ps3000_open_unit@0")(error in=w382, "handle"=w380, "channel"=w379, "coupling"=w378, "range"=w377, "analogueOffset"=w376, "bandwidth"=w373) -> (error out=w381:errorcluster, "PICO_STATUS"=w375:u32, "handle"=w374:i16)  [unwired: 7 in, 1 out]
              }
            }
          }
          frame #5 {
            n48 = To Unsigned Long Integer(number=w400) -> (unsigned 32bit integer=w393:u32)
            n49 = Unbundle By Name(w385) -> ("Enabled"=w394:bool, "Coupling"=w399:i16, "Range"=w398:u16, "Analogue Offset"=w395:dbl, "BandWidth"=w384:u32)
            n50 = Boolean To (0,1)(Boolean=w394) -> (0, 1=w390:i16)
            n51 = To Unsigned Long Integer(number=w399) -> (unsigned 32bit integer=w397:u32)
            n52 = To Unsigned Long Integer(number=w398) -> (unsigned 32bit integer=w396:u32)
            n53 = case shown="False" w394 {
              tunnel: [string ? ("source") string ? ("source")] -> w389
              tunnel: w391 -> [w406 w417]
              tunnel: [w405 w416] -> w388
              tunnel: w392 -> [w404 w415]
              tunnel: w393 -> [w403 w414]
              tunnel: w397 -> [_ w413]
              tunnel: w396 -> [_ w412]
              tunnel: w395 -> [_ w411]
              tunnel: [w402 w410] -> w387
              tunnel: [w401 w409] -> w386
              tunnel: w384 -> [_ w408]
              frame #0 {
                n54 = dll-call lib="ps6000a.dll" fn="ps6000aSetChannelOff" ("ps3000.dll:_ps3000_open_unit@0")(error in=w406, "handle"=w404, "channel"=w403) -> (error out=w405:errorcluster, "PICO_STATUS"=w402:u32, "handle"=w401:i16)  [unwired: 3 in, 1 out]
              }
              frame #1 {
                n55 = dll-call lib="ps6000a.dll" fn="ps6000aSetChannelOn" ("ps3000.dll:_ps3000_open_unit@0")(error in=w417, "handle"=w415, "channel"=w414, "coupling"=w413, "range"=w412, "analogueOffset"=w411, "bandwidth"=w408) -> (error out=w416:errorcluster, "PICO_STATUS"=w410:u32, "handle"=w409:i16)  [unwired: 7 in, 1 out]
              }
            }
          }
          frame #6 {
            n56 = To Unsigned Long Integer(number=w435) -> (unsigned 32bit integer=w428:u32)
            n57 = Unbundle By Name(w420) -> ("Enabled"=w429:bool, "Coupling"=w434:i16, "Range"=w433:u16, "Analogue Offset"=w430:dbl, "BandWidth"=w419:u32)
            n58 = Boolean To (0,1)(Boolean=w429) -> (0, 1=w425:i16)
            n59 = To Unsigned Long Integer(number=w434) -> (unsigned 32bit integer=w432:u32)
            n60 = To Unsigned Long Integer(number=w433) -> (unsigned 32bit integer=w431:u32)
            n61 = case shown="False" w429 {
              tunnel: [string ? ("source") string ? ("source")] -> w424
              tunnel: w426 -> [w441 w452]
              tunnel: [w440 w451] -> w423
              tunnel: w427 -> [w439 w450]
              tunnel: w428 -> [w438 w449]
              tunnel: w432 -> [_ w448]
              tunnel: w431 -> [_ w447]
              tunnel: w430 -> [_ w446]
              tunnel: [w437 w445] -> w422
              tunnel: [w436 w444] -> w421
              tunnel: w419 -> [_ w443]
              frame #0 {
                n62 = dll-call lib="ps6000a.dll" fn="ps6000aSetChannelOff" ("ps3000.dll:_ps3000_open_unit@0")(error in=w441, "handle"=w439, "channel"=w438) -> (error out=w440:errorcluster, "PICO_STATUS"=w437:u32, "handle"=w436:i16)  [unwired: 3 in, 1 out]
              }
              frame #1 {
                n63 = dll-call lib="ps6000a.dll" fn="ps6000aSetChannelOn" ("ps3000.dll:_ps3000_open_unit@0")(error in=w452, "handle"=w450, "channel"=w449, "coupling"=w448, "range"=w447, "analogueOffset"=w446, "bandwidth"=w443) -> (error out=w451:errorcluster, "PICO_STATUS"=w445:u32, "handle"=w444:i16)  [unwired: 7 in, 1 out]
              }
            }
          }
          frame #7 {
            n64 = To Unsigned Long Integer(number=w470) -> (unsigned 32bit integer=w456:u32)
            n65 = Unbundle By Name(w455) -> ("Enabled"=w464:bool, "Coupling"=w469:i16, "Range"=w468:u16, "Analogue Offset"=w465:dbl, "BandWidth"=w454:u32)
            n66 = Boolean To (0,1)(Boolean=w464) -> (0, 1=w463:i16)
            n67 = To Unsigned Long Integer(number=w469) -> (unsigned 32bit integer=w467:u32)
            n68 = To Unsigned Long Integer(number=w468) -> (unsigned 32bit integer=w466:u32)
            n69 = case shown="True" w464 {
              tunnel: [string ? ("source") string ? ("source")] -> w462
              tunnel: w458 -> [w476 w487]
              tunnel: [w475 w486] -> w461
              tunnel: w457 -> [w474 w485]
              tunnel: w456 -> [w473 w484]
              tunnel: w467 -> [_ w483]
              tunnel: w466 -> [_ w482]
              tunnel: w465 -> [_ w481]
              tunnel: [w472 w480] -> w460
              tunnel: [w471 w479] -> w459
              tunnel: w454 -> [_ w478]
              frame #0 {
                n70 = dll-call lib="ps6000a.dll" fn="ps6000aSetChannelOff" ("ps3000.dll:_ps3000_open_unit@0")(error in=w476, "handle"=w474, "channel"=w473) -> (error out=w475:errorcluster, "PICO_STATUS"=w472:u32, "handle"=w471:i16)  [unwired: 3 in, 1 out]
              }
              frame #1 {
                n71 = dll-call lib="ps6000a.dll" fn="ps6000aSetChannelOn" ("ps3000.dll:_ps3000_open_unit@0")(error in=w487, "handle"=w485, "channel"=w484, "coupling"=w483, "range"=w482, "analogueOffset"=w481, "bandwidth"=w478) -> (error out=w486:errorcluster, "PICO_STATUS"=w480:u32, "handle"=w479:i16)  [unwired: 7 in, 1 out]
              }
            }
          }
        }
        n72 = call "PicoStatus.vi"("PICO STATUS"=w201, "error in"=w200, "source"=w199) -> ("error out"=w198:errorcluster)
        n73 = call "PicoErrorHandler2.vi"("error in (no error)"=w198, "handle In"=w197) -> ("error out"=w202:errorcluster)  [unwired: 9 in]
        n74 = Replace Array Subset(array=w204, new element=w205, index=w206) -> (w203:i16[])
      }
      n75 = Unbundle By Name("Trigger Settings") -> ("Trigger Enabled"=w49:bool, "Trigger Source"=w10:u32, "Trigger Threshold (Volts/Probe Units)"=w9:dbl, "Trigger Direction"=w52:u16, "Trigger Delay (samples)"=w51:u64, "Auto Trigger Time (us)"=w50:u32)
      n76 = Unbundle By Name("Digital Channels") -> ("Port 0 Settings"=w21:T6, "Port 1 Settings"=w14:T6)
      n77 = for {
        N: i32 ? -> [_]
        shift-right: [w106] -> w18
        shift-left: w20 -> [w110]
        shift-right: [w102] -> w17
        shift-left: w19 -> [w111]
        shift-right: [w107] -> w24
        shift-left: w23 -> [w108]
        tunnel: w21 -> [w100]
        tunnel: i32 ? -> [w97]
        tunnel: w14 -> [w95]
        i -> [w96]
        n78 = Add(x=w96, y=w97) -> (x+y=w98:i32)
        n79 = case shown="0" w96 {
          tunnel: w111 -> [w119 w149 w187]
          tunnel: w110 -> [w125 w151 w188]
          tunnel: [w127 w163 i16 ?] -> w109
          tunnel: [w122 w160 u32 ? ("PICO_STATUS")] -> w105
          tunnel: [w124 w161 w188] -> w104
          tunnel: [w126 w162 string ? ("source")] -> w103
          tunnel: [w121 w159 w187] -> w102
          tunnel: w100 -> [w116 _ _]
          tunnel: w98 -> [w118 w158 _]
          tunnel: w95 -> [_ w157 _]
          frame #0 {
            n80 = Unbundle By Name(w116) -> ("Enabled"=w120:bool, "Threshold Level (Volts)"=w115:dbl[], "Hysteresis"=w117:u32)
            n81 = To Unsigned Long Integer(number=w118) -> (unsigned 32bit integer=w123:u32)
            n82 = for {
              tunnel: w115 -> [w130] mode=indexing
              tunnel: [w129] -> w114 mode=indexing
              # "5V is range 8"
              n83 = call "PicoScopeVoltsToAdc.vi"("Volts"=w130, "Range Index"=u16 ?) -> ("ADC count"=w129:i16)  [unwired: 1 in]
            }
            n84 = Array Size(array=w114) -> (size(s)=w112:i32)
            n85 = To Word Integer(number=w112) -> (16bit integer=w113:i16)
            n86 = Boolean To (0,1)(Boolean=w120) -> (0, 1=w127:i16)
            n87 = case shown="True" w120 {
              tunnel: [string ? ("source") string ? ("source")] -> w126
              tunnel: w125 -> [w136 w146]
              tunnel: [w135 w145] -> w124
              tunnel: w123 -> [w134 w144]
              tunnel: w114 -> [_ w143]
              tunnel: w113 -> [_ w142]
              tunnel: w117 -> [_ w139]
              tunnel: [w133 w141] -> w122
              tunnel: [w132 w140] -> w121
              tunnel: w119 -> [w131 w138]
              frame #0 {
                n88 = dll-call lib="ps6000a.dll" fn="ps6000aSetDigitalPortOff" ("ps3000.dll:_ps3000_open_unit@0")(error in=w136, "handle"=w131, "port"=w134) -> (error out=w135:errorcluster, "PICO_STATUS"=w133:u32, "handle"=w132:i16)  [unwired: 3 in, 1 out]
              }
              frame #1 {
                n89 = dll-call lib="ps6000a.dll" fn="ps6000aSetDigitalPortOn" ("ps3000.dll:_ps3000_open_unit@0")(error in=w146, "handle"=w138, "port"=w144, "logicThresholdLevel"=w143, "logicThresholdLevelLength"=w142, "hysteresis"=w139) -> (error out=w145:errorcluster, "PICO_STATUS"=w141:u32, "handle"=w140:i16)  [unwired: 6 in, 1 out]
              }
            }
          }
          frame #1 {
            n90 = Unbundle By Name(w157) -> ("Enabled"=w152:bool, "Threshold Level (Volts)"=w148:dbl[], "Hysteresis"=w155:u32)
            n91 = To Unsigned Long Integer(number=w158) -> (unsigned 32bit integer=w150:u32)
            n92 = for {
              tunnel: w148 -> [w166] mode=indexing
              tunnel: [w165] -> w153 mode=indexing
              # "5V is range 8"
              n93 = call "PicoScopeVoltsToAdc.vi"("Volts"=w166, "Range Index"=u16 ?) -> ("ADC count"=w165:i16)  [unwired: 1 in]
            }
            n94 = Boolean To (0,1)(Boolean=w152) -> (0, 1=w163:i16)
            n95 = Array Size(array=w153) -> (size(s)=w156:i32)
            n96 = To Word Integer(number=w156) -> (16bit integer=w154:i16)
            n97 = case shown="True" w152 {
              tunnel: [string ? ("source") string ? ("source")] -> w162
              tunnel: w151 -> [w172 w182]
              tunnel: [w171 w181] -> w161
              tunnel: w150 -> [w170 w180]
              tunnel: w153 -> [_ w179]
              tunnel: w154 -> [_ w178]
              tunnel: w155 -> [_ w175]
              tunnel: [w169 w177] -> w160
              tunnel: [w168 w176] -> w159
              tunnel: w149 -> [w167 w174]
              frame #0 {
                n98 = dll-call lib="ps6000a.dll" fn="ps6000aSetDigitalPortOff" ("ps3000.dll:_ps3000_open_unit@0")(error in=w172, "handle"=w167, "port"=w170) -> (error out=w171:errorcluster, "PICO_STATUS"=w169:u32, "handle"=w168:i16)  [unwired: 3 in, 1 out]
              }
              frame #1 {
                n99 = dll-call lib="ps6000a.dll" fn="ps6000aSetDigitalPortOn" ("ps3000.dll:_ps3000_open_unit@0")(error in=w182, "handle"=w174, "port"=w180, "logicThresholdLevel"=w179, "logicThresholdLevelLength"=w178, "hysteresis"=w175) -> (error out=w181:errorcluster, "PICO_STATUS"=w177:u32, "handle"=w176:i16)  [unwired: 6 in, 1 out]
              }
            }
          }
          frame #2 {
          }
        }
        n100 = call "PicoStatus.vi"("PICO STATUS"=w105, "error in"=w104, "source"=w103) -> ("error out"=w99:errorcluster)
        n101 = Add(x=w96, y=i32 ?) -> (x+y=w94:i32)
        n102 = call "PicoErrorHandler2.vi"("error in (no error)"=w99, "handle In"=w102) -> ("error out"=w106:errorcluster)  [unwired: 9 in]
        n103 = Replace Array Subset(array=w108, new element=w109, index=w94) -> (w107:i16[])
      }
      "Enabled array" <- w24
      n104 = local read "Channels"() -> (w13:T2)
      n105 = case shown="1001" w10 {
        tunnel: [w59 w63 w67 w71 w75 w79 w83 w87 u16 ? ("Range") u16 ? ("Range") u16 ? ("Range")] -> w8
        tunnel: w13 -> [w58 w62 w66 w70 w74 w78 w82 w86 _ _ _]
        tunnel: w9 -> [w56 w60 w64 w68 w72 w76 w80 w84 w88 w90 _]
        tunnel: [w56 w60 w64 w68 w72 w76 w80 w84 w88 w90 dbl ? ("Trigger Threshold (Volts/Probe Units)")] -> w7
        frame #0 {
          n106 = Unbundle By Name(w58) -> ("Channel A Settings"=w57:T5)  [unwired: 7 out]
          n107 = Unbundle By Name(w57) -> ("Range"=w59:u16)
        }
        frame #1 {
          n108 = Unbundle By Name(w62) -> ("Channel B Settings"=w61:T5)  [unwired: 7 out]
          n109 = Unbundle By Name(w61) -> ("Range"=w63:u16)
        }
        frame #2 {
          n110 = Unbundle By Name(w66) -> ("Channel C Settings"=w65:T5)  [unwired: 7 out]
          n111 = Unbundle By Name(w65) -> ("Range"=w67:u16)
        }
        frame #3 {
          n112 = Unbundle By Name(w70) -> ("Channel D Settings"=w69:T5)  [unwired: 7 out]
          n113 = Unbundle By Name(w69) -> ("Range"=w71:u16)
        }
        frame #4 {
          n114 = Unbundle By Name(w74) -> ("Channel E Settings"=w73:T5)  [unwired: 7 out]
          n115 = Unbundle By Name(w73) -> ("Range"=w75:u16)
        }
        frame #5 {
          n116 = Unbundle By Name(w78) -> ("Channel F Settings"=w77:T5)  [unwired: 7 out]
          n117 = Unbundle By Name(w77) -> ("Range"=w79:u16)
        }
        frame #6 {
          n118 = Unbundle By Name(w82) -> ("Channel G Settings"=w81:T5)  [unwired: 7 out]
          n119 = Unbundle By Name(w81) -> ("Range"=w83:u16)
        }
        frame #7 {
          n120 = Unbundle By Name(w86) -> ("Channel H Settings"=w85:T5)  [unwired: 7 out]
          n121 = Unbundle By Name(w85) -> ("Range"=w87:u16)
        }
        frame #8 {
          # "Trigger Port 0"
        }
        frame #9 {
          # "Trigger Port 1"
        }
        frame #10 {
          # "Not Adjustable has a Fixed threshold of 1.25 V"
          # "Trigger AUX"
        }
      }
      n122 = To Unsigned Long Integer(number=w10) -> (unsigned 32bit integer=w55:u32)
      n123 = Boolean To (0,1)(Boolean=w49) -> (0, 1=w48:i16)
      n124 = To Unsigned Long Integer(number=w52) -> (unsigned 32bit integer=w54:u32)
      n125 = call "PicoScopeVoltsToAdc.vi"("Max_adc"="Max ADC value", "Volts"=w7, "Range Index"=w8) -> ("ADC count"=w11:i16)
      n126 = dll-call lib="ps6000a.dll" fn="ps6000aSetSimpleTrigger" ("ps3000.dll:_ps3000_open_unit@0")(error in=w18, "handle"=w17, "enable"=w48, "source"=w55, "threshold"=w11, "direction"=w54, "delay"=w51, "autoTrigger_us"=w50) -> (error out=w46:errorcluster, "PICO_STATUS"=w47:u32, "handle"=w34:i16)  [unwired: 8 in, 1 out]
      n127 = call "PicoStatus.vi"("PICO STATUS"=w47, "error in"=w46, "source"=string ?) -> ("error out"=w35:errorcluster)
      n128 = call "PicoErrorHandler2.vi"("error in (no error)"=w35, "handle In"=w34) -> ("error out"=w36:errorcluster)  [unwired: 9 in]
    }
    frame #1 {
    }
  }
  "error out" <- w5
  "handle out" <- w6
